vi "SafeIntakeMode.vi"() -> (0 "Rollers Active?":bool, 1 "Angle Power":dbl, 3 "Roller Power":dbl)   [LabVIEW 2015]
uses:
  Common Code/Intake States.ctl
  Common Code/Intake Commands.ctl
  Robot Global Data.vi
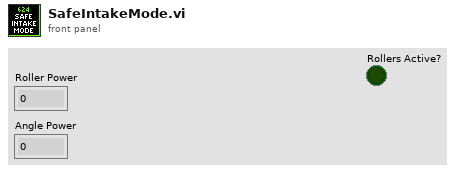
[diagram p1: front panel]
types:
  T1 = typedef "Intake States.ctl" = enum16{"Idle", "Set roller speed", "Move to angle", "Go Hard or Go Home", "Ball Settle"}
  T2 = typedef "Dashboard Control Data.ctl" = cluster{"Encoder Control":T3, "Steer PID output":cluster{"output high":dbl, "output low":dbl}, " Steer PID gains":cluster{"proportional gain (Kc)":dbl, "integral time (Ti, min)":dbl, "derivative time (Td, min)":dbl}, "Drivetrain Settings":T4, "Vision Packet":T5, "Dashboard Drivetrain Command":T6, "Info/Command Cluster":T8, "Ball Vision Packet":T9, "Intake Presets":T11, "Intake Encoder Control":T13, "Climb Presets":T14, "Goal Output Range":cluster{"output high":dbl, "output low":dbl}, "Enabled Systems":T15, "Auton Presets":T16, "Pressure M":dbl, "Pressure B":dbl, "Vision Timeout":dbl, "Auto-Shift":T17, "Catapult Setpoints":T18}
  T3 = typedef "Encoder Control.ctl" = cluster{"Right Tick Constant":dbl, "Left Tick Constant":dbl, "Reset?":bool, "Y Dist":cluster{"PID gains":cluster{"proportional gain (Kc)":dbl, "integral time (Ti, min)":dbl, "derivative time (Td, min)":dbl}}, "Y Stop Thresh":dbl, "Y Stop Speed":dbl}
  T4 = typedef "Drivetrain Settings.ctl" = cluster{"Gyro Tolerance":dbl, "Throttle Ramp (ms)":dbl, "Kv":dbl, "Ka":dbl, "Feed Forward P":dbl, "Feed Forward D":dbl, "Goal Vision PID gains":cluster{"proportional gain (Kc)":dbl, "integral time (Ti, min)":dbl, "derivative time (Td, min)":dbl}, "Goal Detection Window":dbl, "Creep Rate":dbl, "Vision Throttle Threshold":dbl, "Min Turn Output":dbl, "Left Batter Angle":dbl, "Right Batter Angle":dbl}
  T5 = typedef "Goal Vision Packet.ctl" = cluster{"Distance":dbl, "Center X":dbl, "Center Y":dbl, "Found Target?":bool, "Robot Center":dbl, "Angle":dbl}
  T6 = typedef "Dashboard Drivetrain Command.ctl" = cluster{"Drivetrain Vision":T7}
  T7 = typedef "Drivetrain Vision.ctl" = cluster{"Goal Window":dbl, "Ball Window":dbl}
  T8 = typedef "Ball Tracking Command Cluster.ctl" = cluster{"Distance to Ball":dbl, "Desired Angle":dbl, "Command":enum16{"Turn to Ball", "Turn to Angle", "Get Distance"}, "Pixels from Center":dbl}
  T9 = typedef "Ball Vision Packet.ctl" = cluster{"Ball Detected?":bool, "Distance to Ball":dbl, "Desired Angle":dbl, "Pixels from Center":dbl, "Tracking mode":T10}
  T10 = typedef "Tracking Mode.ctl" = enum16{"Turn to Ball", "Turn to Angle"}
  T11 = typedef "Intake Presets.ctl" = cluster{"Intake Speed":dbl, "Outake Speed":dbl, "Low Height":dbl, "Half Height":dbl, "High Idle Height":dbl, "Angle Speed":dbl, "Angle Tolerance":dbl, "Encoder Scale":dbl, "Load Height":dbl, "Output Range":T12, "Rotation Power Max/Min":dbl, "MaxCurrent":dbl, "Intake Trip Time":dbl, "Idle Height":dbl, "Max Height":dbl, "Reset Encoders?":bool, "PID gains":cluster{"proportional gain (Kc)":dbl, "integral time (Ti, min)":dbl, "derivative time (Td, min)":dbl}, "Intake Stop Delay":u32, "Settle Time":dbl, "Settle Wait Time":dbl, "Pull Up Delay":dbl}
  T12 = typedef "Drivetrain Output Range.ctl" = cluster{"output high":dbl, "output low":dbl}
  T13 = typedef "IntakeEcoderControl.ctl" = cluster{"Arm Tick Constant":dbl, "Reset?":bool, "Y Dist":cluster{"PID gains":cluster{"proportional gain (Kc)":dbl, "integral time (Ti, min)":dbl, "derivative time (Td, min)":dbl}}, "Y Stop Thresh":dbl, "Y Stop Speed":dbl}
  T14 = typedef "Climb Presets.ctl" = cluster{"Pull Power":dbl, "Extend Power":dbl}
  T15 = typedef "Enabled Systems.ctl" = cluster{"Shoot":bool, "Intake":bool, "DT":bool, "Gyro":bool, "100ms":bool, "US":bool}
  T16 = typedef "Autonomous Presets.ctl" = cluster{"Pitch Limit":dbl, "Roll Limit":dbl, "Start Position":dbl, "Cross Position":dbl}
  T17 = typedef "Auto Shift Cluster.ctl" = cluster{"Delay":dbl, "Speed Thresh":dbl, "Upshift Accel":dbl, "Upshift Throttle":dbl, "Upshift Throttle Accel":dbl, "Downshift Throttle":dbl, "Downshift Throttle Accel":dbl, "Pressure Threshold":dbl}
  T18 = typedef "Catapult Presets.ctl" = cluster{"Intake Danger Height":dbl, "Ball Security Delay ":dbl, "High PSI Minimum":dbl, "Shot Finish Delay":dbl, "Low PSI Minimum":dbl, "Idle Ball Security Wait ":dbl}
  T19 = typedef "Intake Commands Cluster.ctl" = cluster{"Intake Commands":T20, "Intake Mode":T21, "Override IR":bool, "Angle Target":dbl}
  T20 = typedef "Intake Commands.ctl" = enum16{"Settle Ball", "Unload", "Load", "Pull up", "Drop low", "Idle", "Lift Half", "Go To Angle"}
  T21 = typedef "Intake Mode.ctl" = enum16{"Safe", "Auto", "Manual"}
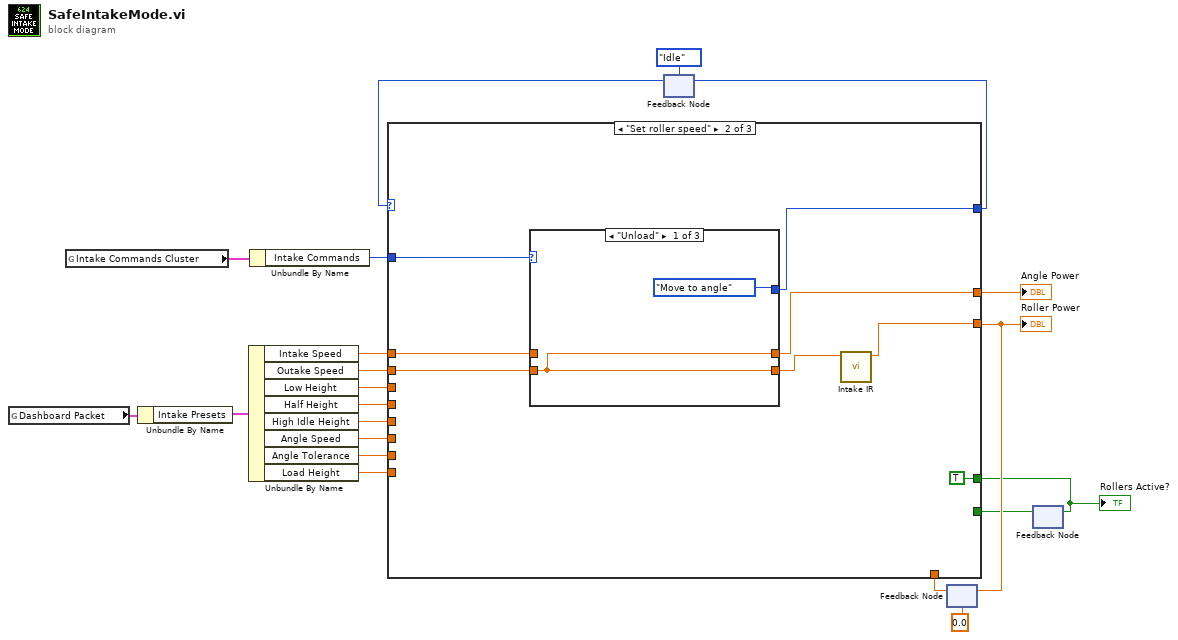
[diagram p0: block diagram]
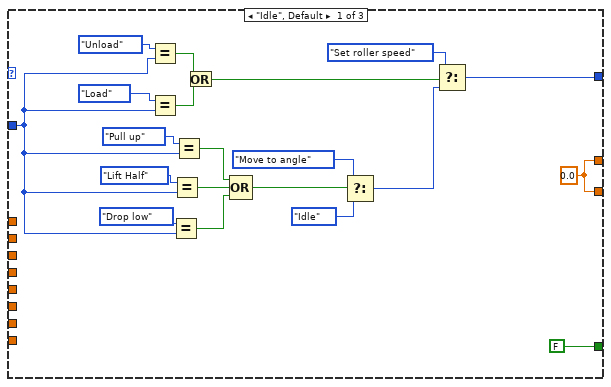
[diagram p2: hidden frame]
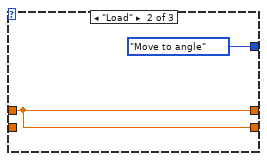
[diagram p3: hidden frame]
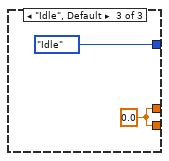
[diagram p4: hidden frame]
diagram:
  n1 = global read "Robot Global Data.vi" "Dashboard Packet"() -> (w21:T2)
  n2 = global read "Robot Global Data.vi" "Intake Commands Cluster"() -> (w7:T19)
  n3 = Unbundle By Name(w21) -> ("Intake Presets"=w20:T11)
  n4 = Unbundle By Name(w20) -> ("Intake Speed"=w19:dbl, "Outake Speed"=w18:dbl, "Low Height"=w17:dbl, "Half Height"=w16:dbl, "High Idle Height"=w15:dbl, "Angle Speed"=w14:dbl, "Angle Tolerance"=w13:dbl, "Load Height"=w6:dbl)
  n5 = Unbundle By Name(w7) -> ("Intake Commands"=w12:T20)
  n6 = feedback #1(Intake_States."Idle" ("Intake States")) -> (w11:T1)
  n7 = feedback #2(0.0 ("Intake Speed")) -> (w8:dbl)
  n8 = feedback #3() -> (w1:bool)  [unwired: 1 in]
  n9 = case shown="\"Set roller speed\"" w11 {
    tunnel: w19 -> [_ w49 _]
    tunnel: w18 -> [_ w48 _]
    tunnel: w17 -> [_ _ _]
    tunnel: w16 -> [_ _ _]
    tunnel: w15 -> [_ _ _]
    tunnel: w14 -> [_ _ _]
    tunnel: w13 -> [_ _ _]
    tunnel: w12 -> [w23 w46 _]
    tunnel: [w25 w47 _] -> w10
    tunnel: [w24 w42 w57] -> w4
    tunnel: w8 -> [_ _ w57]
    tunnel: w6 -> [_ _ _]
    tunnel: [w24 w45 _] -> w5
    tunnel: [FALSE TRUE w56] -> w2
    tunnel: w1 -> [_ _ w56]
    frame "Idle", Default {
      w24 = 0.0
      n10 = Equal?(x=Intake_Commands."Unload" ("Intake Commands"), y=w23) -> (x = y?=w39:bool)
      n11 = Equal?(x=Intake_Commands."Load" ("Intake Commands"), y=w23) -> (x = y?=w38:bool)
      n12 = Equal?(x=Intake_Commands."Drop low" ("Intake Commands"), y=w23) -> (x = y?=w32:bool)
      n13 = Equal?(x=Intake_Commands."Lift Half" ("Intake Commands"), y=w23) -> (x = y?=w33:bool)
      n14 = Equal?(x=Intake_Commands."Pull up" ("Intake Commands"), y=w23) -> (x = y?=w34:bool)
      n15 = Or(x=w39, y=w38) -> (x .or. y?=w31:bool)
      n16 = Compound Arithmetic op=OR(w34, w33, w32) -> (w29:bool)
      n17 = Select(t=Intake_States."Move to angle" ("Intake States"), s=w29, f=Intake_States."Idle" ("Intake States")) -> (s? t:f=w26:T1)
      n18 = Select(t=Intake_States."Set roller speed" ("Intake States"), s=w31, f=w26) -> (s? t:f=w25:T1)
    }
    frame "Set roller speed" {
      n19 = case shown="\"Unload\"" w46 {
        tunnel: w49 -> [_ w52 _]
        tunnel: w48 -> [w50 _ _]
        tunnel: [w50 w52 w54] -> w43
        tunnel: [Intake_States."Move to angle" ("Intake States") Intake_States."Move to angle" ("Intake States") Intake_States."Idle" ("Intake States")] -> w47
        tunnel: [w50 w52 w54] -> w45
        frame "Unload" {
        }
        frame "Load" {
        }
        frame "Idle", Default {
          w54 = 0.0 ("Intake Speed")
        }
      }
      n20 = call "Intake IR.vi"("Speed"=w43) -> ("Speeeeeeed"=w42:dbl)  [unwired: 9 in, 1 out]
    }
    frame "Move to angle" {
    }
  }
  "Angle Power" <- w5
  "Roller Power" <- w4
  "Rollers Active?" <- w2
  n21 = feedback-in #1(w10) -> ()
  n22 = feedback-in #2(w4) -> ()
  n23 = feedback-in #3(w2) -> ()
